vi "Sort Channels By Offset.vi"(8 "error in (no error)":errorcluster, 11 "Transfer Configuration in":refnum<class "Configuration.Transfer.lvclass">) -> (0 "error out":errorcluster, 3 "Transfer Configuration out":refnum<class "Configuration.Transfer.lvclass">)   [LabVIEW 2016, in "Configuration.Transfer.lvclass"]
uses:
  Configuration.Transfer.lvclass
  Configuration.Transfer.lvclass/Configuration.Transfer.ctl
  Configuration.Channel/Configuration.Channel.lvclass/Configuration.Channel.ctl
  Configuration.Channel/Configuration.Channel.lvclass
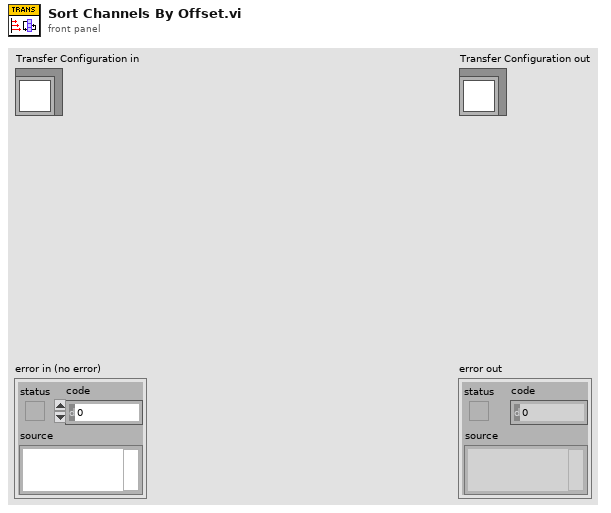
[diagram p1: front panel]
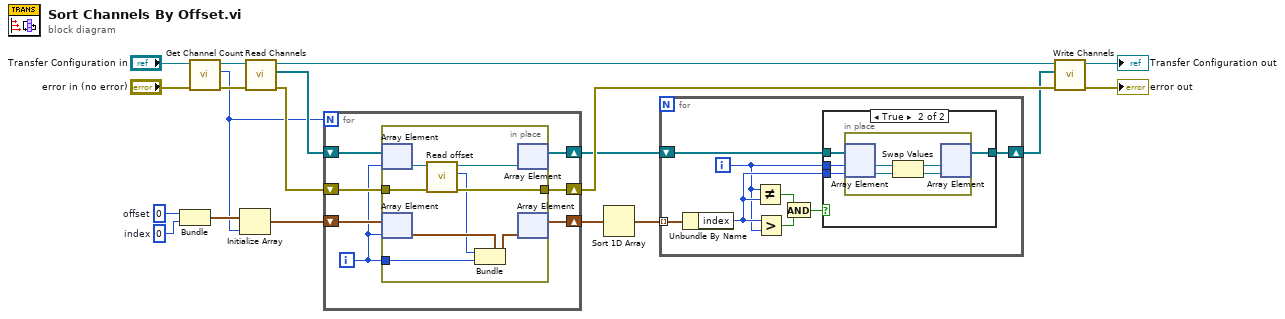
[diagram p0: block diagram]
diagram:
  w16 = 0  # index
  w17 = u64 0  # offset
  n1 = Bundle("offset"=w17, "index"=w16) -> (w15:cluster{"offset":u64, "index":i32})  [unwired: 1 in]
  n2 = call "Get Channel Count.vi"("error in (no error)"="error in (no error)", "Transfer Configuration in"="Transfer Configuration in") -> ("error out"=w13:errorcluster, "channel count"=w8:i32, "Transfer Configuration out"=w14:refnum<class "Configuration.Transfer.lvclass">)  [unwired: 7 in]
  n3 = Initialize Array(w15, w8) -> (w11:cluster{"offset":u64, "index":i32}[])
  n4 = call "Read Channels.vi"("error in (no error)"=w13, "Configuration.Transfer in"=w14) -> ("error out"=w10:errorcluster, "Channels"=w12:refnum<class "Configuration.Channel.lvclass">[], "Configuration.Transfer out"=w6:refnum<class "Configuration.Transfer.lvclass">)  [unwired: 7 in]
  n5 = for {
    N: w8 -> [_]
    shift-right: [w22] -> w3
    shift-left: w10 -> [w23]
    shift-right: [w25] -> w9
    shift-left: w11 -> [w26]
    shift-right: [w20] -> w2
    shift-left: w12 -> [w24]
    i -> [w21]
    n6 = in-place {
      in-place-border: w21 -> [w34]
      in-place-border: w23 -> [w29]
      in-place-border: [w28] -> w22
      n7 = in-place-array #1(w24, w21) -> (w31:refnum<class "Configuration.Channel.lvclass">)
      n8 = in-place-array #2(w26, w21) -> (w33:cluster{"offset":u64, "index":i32})
      n9 = call "Read offset.vi"("error in (no error)"=w29, "Configuration.Channel in"=w31) -> ("error out"=w28:errorcluster, "offset"=w27:u64, "Configuration.Channel out"=w30:refnum<class "Configuration.Channel.lvclass">)  [unwired: 7 in]
      n10 = Bundle(cluster=w33, "offset"=w27, "index"=w34) -> (w32:cluster{"offset":u64, "index":i32})
      n11 = in-place-array #1(w30) -> (w20:refnum<class "Configuration.Channel.lvclass">[])  [unwired: 1 out]
      n12 = in-place-array #2(w32) -> (w25:cluster{"offset":u64, "index":i32}[])  [unwired: 1 out]
    }
  }
  n13 = Sort 1D Array(array=w9) -> (sorted array=w7:cluster{"offset":u64, "index":i32}[])
  n14 = for {
    shift-right: [w41] -> w1
    shift-left: w2 -> [w42]
    tunnel: w7 -> [w40] mode=indexing
    i -> [w38]
    n15 = Unbundle By Name(w40) -> ("index"=w39:i32)
    n16 = Not Equal?(x=w38, y=w39) -> (x != y?=w37:bool)
    n17 = Greater?(x=w39, y=w38) -> (0:w36:bool)
    n18 = And(x=w37, y=w36) -> (x .and. y?=w35:bool)
    n19 = case shown="True" w35 {
      tunnel: w42 -> [w43 w47]
      tunnel: [w43 w46] -> w41
      tunnel: w38 -> [_ w45]
      tunnel: w39 -> [_ w44]
      frame False {
      }
      frame True {
        n20 = in-place {
          n21 = in-place-array #3(w47, w45, w44) -> (w51:refnum<class "Configuration.Channel.lvclass">, w50:refnum<class "Configuration.Channel.lvclass">)
          n22 = Swap Values(12:w51, 14:w50) -> (1:w49:refnum<class "Configuration.Channel.lvclass">, 3:w48:refnum<class "Configuration.Channel.lvclass">)  [unwired: 1 in]
          n23 = in-place-array #3(w49, w48) -> (w46:refnum<class "Configuration.Channel.lvclass">[])  [unwired: 2 out]
        }
      }
    }
  }
  n24 = call "Write Channels.vi"("error in (no error)"=w3, "Channels"=w1, "Configuration.Transfer in"=w6) -> ("error out"=→"error out":errorcluster, "Configuration.Transfer out"=→"Transfer Configuration out":refnum<class "Configuration.Transfer.lvclass">)  [unwired: 7 in]
